vi "Read Stop Event.vi"(11 "IEventHandler in":refnum<class "IEventHandler.lvclass">) -> (2 "Stop! Event":refnum<user-event>)   [LabVIEW 2015, in "ActorEvents.lvlib" / "IEventHandler.lvclass"]
uses:
  IEventHandler.lvclass
  IEventHandler.lvclass/IEventHandler.ctl
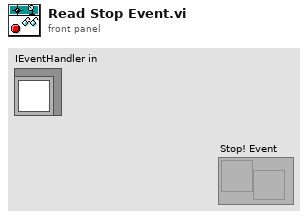
[diagram p1: front panel]
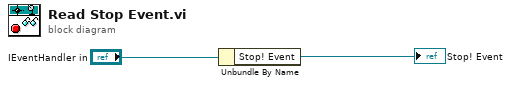
[diagram p0: block diagram]
diagram:
  n1 = Unbundle By Name("IEventHandler in") -> ("Stop! Event"=→"Stop! Event":refnum<user-event>)
